vi "CheckInOpened.vi"(8 "error in (no error)":errorcluster, 10 "GUID":string, 11 "SMO.UI.MAUI in":refnum<class "SMO.UI.MAUI.lvclass">) -> (0 "error out":errorcluster, 1 "Index":i32, 2 "InOpened?":bool, 3 "SMO.UI.MAUI out":refnum<class "SMO.UI.MAUI.lvclass">)   [LabVIEW 2019, in "SMO.UI.MAUI.lvclass"]
doc: "Checks if a subpanel is in \"Opened\" category of the class data based on the SMO GUID. Originally created for the Open Panel method which has been sidelined for now due to issues in LabVIEW."
uses:
  SMO.UI.MAUI.lvclass
  SMO.UI.MAUI.lvclass/SMO.UI.MAUI.ctl
  <userlib>/LevyLab/Embedded UI/SMO.UI.Embedded/SMO.UI.Embedded.lvclass
  C:/Program Files (x86)/National Instruments/LabVIEW 2019/vi.lib/JKI/JKI SMO/SMO/SMO.lvclass
  <vilib>/JKI/JKI SMO/SMO/SMO.lvclass
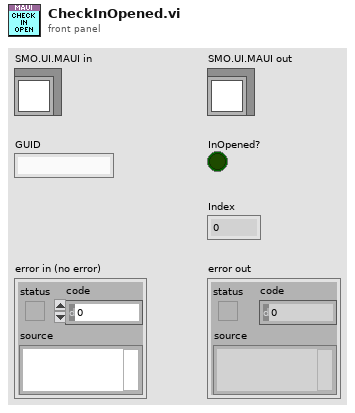
[diagram p1: front panel]
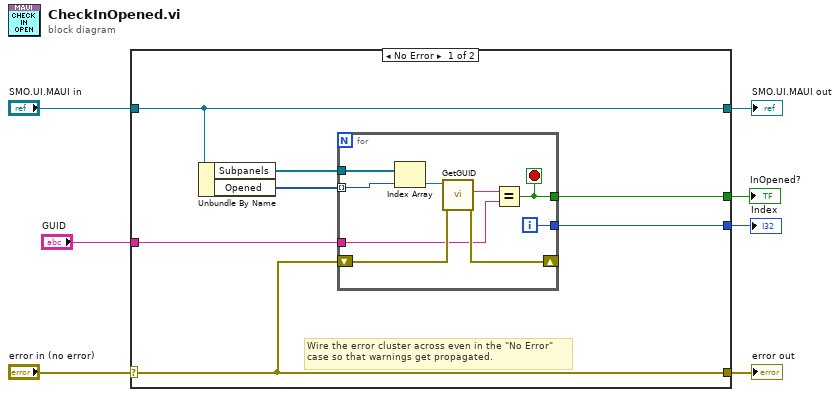
[diagram p0: block diagram]
diagram:
  n1 = case shown="No Error" "error in (no error)" {
    selector: "error in (no error)" -> [w14 w25]
    tunnel: [w14 w25] -> w6
    tunnel: [w13 w24] -> w4
    tunnel: "SMO.UI.MAUI in" -> [w13 w24]
    tunnel: "GUID" -> [w10 _]
    tunnel: [w9 _] -> w2
    tunnel: [w8 _] -> w1
    frame No Error {
      # "Wire the error cluster across even in the \"No Error\"\ncase so that warnings get propagated."
      n2 = Unbundle By Name(w13) -> ("Subpanels"=w12:refnum<class "SMO.UI.Embedded.lvclass">[], "Opened"=w11:i32[])
      n3 = for {
        tunnel: w12 -> [w21]
        tunnel: w11 -> [w16] mode=indexing
        tunnel: w10 -> [w18]
        shift-right: [w22] -> _
        shift-left: w14 -> [w23]
        tunnel: [w17] -> w9
        tunnel: [w15] -> w8
        i -> [w15]
        stop <- w17 stop-if-true
        n4 = Index Array(array=w21, index=w16) -> (element=w20:refnum<class "SMO.UI.Embedded.lvclass">)
        n5 = call <vilib>:"GetGUID.vi"("error in (no error)"=w23, "SMO"=w20) -> ("error out"=w22:errorcluster, "GUID"=w19:string)  [unwired: 7 in, 1 out]
        n6 = Equal?(x=w19, y=w18) -> (x = y?=w17:bool)
      }
    }
    frame Error {
    }
  }
  "error out" <- w6
  "SMO.UI.MAUI out" <- w4
  "InOpened?" <- w2
  "Index" <- w1
